vi "MDML_disconnect.vi"(8 "error in (no error)":errorcluster) -> (0 "error out":errorcluster)   [LabVIEW 2018]
uses:
  Downloads/mqtt_lv2013_201708181938/mqtt_lv2013/mqtt Folder/src/class/mqtt/mqttTXqueue/mqttTXdataQueueFunction.ctl
  Downloads/mqtt_lv2013_201708181938/mqtt_lv2013/mqtt Folder/src/class/mqtt/mqttTXqueue/mqttRXsubscriptionEventFunction.ctl
  Downloads/mqtt_lv2013_201708181938/mqtt_lv2013/mqtt Folder/src/class/mqtt/mqtt.lvclass
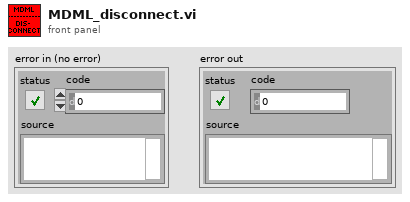
[diagram p1: front panel]
types:
  T1 = typedef "mqttRXsubscriptionEventFunction.ctl" = enum16{"init", "deinit", "getEventRef", "event"}
  T2 = typedef "mqttTXdataQueueFunction.ctl" = enum16{"init", "deinit", "getQueue", "enqueue"}
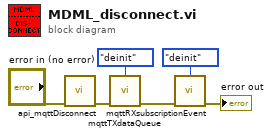
[diagram p0: block diagram]
diagram:
  n1 = call "api_mqttDisconnect.vi"("error in (no error)"="error in (no error)") -> ("error out"=w2:errorcluster)  [unwired: 13 in, 1 out]
  n2 = call "mqttTXdataQueue.vi"("function"=mqttTXdataQueueFunction."deinit", "error in (no error)"=w2) -> ("error out"=w4:errorcluster)  [unwired: 12 in, 1 out]
  n3 = call "mqttRXsubscriptionEvent.vi"("function"=mqttRXsubscriptionEventFunction."deinit", "error in (no error)"=w4) -> ("error out"=→"error out":errorcluster)  [unwired: 12 in, 1 out]
